vi "prepare_smith_plot.vi"(5 "left_center":dbl=300.0, 7 "top_center":dbl=300.0, 8 "x_scale":bool=TRUE, 9 "r_scale":bool=TRUE, 10 "dimensions (w,h)":cluster{"width":i16, "height":i16}={"width"=600, "height"=600}, 11 "smith plot":cluster{"r":dbl, "x":dbl}[](array[cluster])=[{"r"=2.0, "x"=2.0}, {"r"=4.0, "x"=-2.0}] {"x" format="%0.2f"; "r" format="%0.2f"}) -> (3 "smith_out":picture)   [LabVIEW 2025]
uses:
  <vilib>/picture/smith.llb/Smith Plot Style.ctl
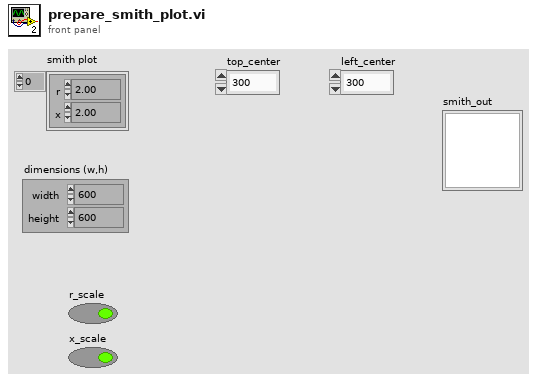
[diagram p1: front panel]
types:
  T1 = cluster{"Width":u16, "Style":enum32{"Solid", "Dash", "Dot", "DashDot", "DashDotDot"}}
  T2 = typedef "Smith Plot Style.ctl" = u16
  T3 = cluster{"Plot Style":T2, "Line Color":u32, "Point Color":u32}
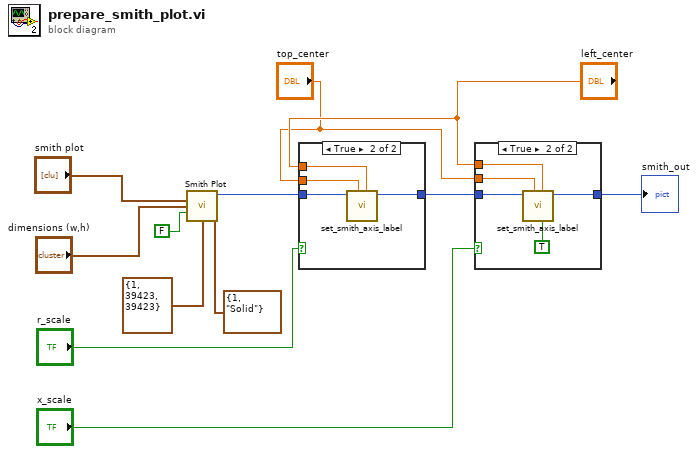
[diagram p0: block diagram]
diagram:
  n1 = call <vilib>:"Smith Plot.vi"("smith plot"="smith plot", "dimensions (w,h)"="dimensions (w,h)", "dimensions incl scales? (T)"=FALSE, "smith plot cosmetics"=T3 {"Plot Style"=1, "Line Color"=39423, "Point Color"=39423}, "Pen Cosmetics"=T1 {"Width"=1, "Style"=enum."Solid"}) -> ("new picture"=w11:picture)  [unwired: 10 in]
  n2 = case shown="True" "r_scale" {
    tunnel: w11 -> [w13 w17]
    tunnel: [w13 w16] -> w9
    tunnel: "top_center" -> [_ w15]
    tunnel: "left_center" -> [_ w14]
    frame False {
    }
    frame True {
      n3 = call "set_smith_axis_label.vi"("left_center"=w14, "top_center"=w15, "smith_in"=w17) -> ("smith_out"=w16:picture)  [unwired: 8 in]
    }
  }
  n4 = case shown="True" "x_scale" {
    tunnel: w9 -> [w18 w22]
    tunnel: "left_center" -> [_ w21]
    tunnel: "top_center" -> [_ w20]
    tunnel: [w18 w19] -> w2
    frame False {
    }
    frame True {
      n5 = call "set_smith_axis_label.vi"("r/x_scale"=TRUE, "left_center"=w21, "top_center"=w20, "smith_in"=w22) -> ("smith_out"=w19:picture)  [unwired: 7 in]
    }
  }
  "smith_out" <- w2
